vi "remote.Log In.vi"(0 "SLSC Remote in":refnum<class "SLSC Interface.lvclass">, 1 "username":string, 2 "password":string, 5 "chassis":refnum<k21>, 11 "error in (no error)":errorcluster, 12 "connect timeout (60 sec)":dbl=60.0, 13 "save credentials to disk? (F)":bool) -> (4 "SLSC Remote out":refnum<class "SLSC Interface.lvclass">, 15 "error out":errorcluster)   [LabVIEW 2016, in "SLSC Interfaces.lvlib" / "SLSC Interface.lvclass"]
uses:
  SLSC Interface Class/SLSC Interface.lvclass
  SLSC Interface Class/SLSC Interface.lvclass/SLSC Interface.ctl
  SLSC Interface Class/Read client handle.vi
  SLSC Interface Class/Read URL.vi
  <vilib>/NI/JSON Support for LabVIEW/JSON Data Classes/JSON Object/JSON Object.lvclass
  C:/Program Files (x86)/National Instruments/LabVIEW 2016/vi.lib/NI/JSON Support for LabVIEW/JSON Data Classes/JSON Datatype/JSON Null.lvclass
  SLSC Interface Class/Read session.vi
  <vilib>/NI/JSON Support for LabVIEW/JSON Data Classes/JSON Object/New JSON Object (Empty).vi
  <vilib>/NI/JSON Support for LabVIEW/JSON Data Classes/JSON Object/Insert Key Value Pair (Single String).vi
  <vilib>/NI/JSON Support for LabVIEW/JSON Data Classes/JSON Object/Insert Key Value Pair (Single Numeric).vi
  <vilib>/NI/JSON Support for LabVIEW/JSON Data Classes/JSON Object/Insert Key Value Pair (Single Boolean).vi
  <vilib>/NI/NI JSONRPC Server Framework/Classes/Server/Format Client Request (Auto-Increment).vi
  <vilib>/httpClient/POSTBuffer.vi
  <vilib>/NI/NI JSONRPC Server Framework/Classes/Server/Parse Response (Object).vi
  <vilib>/NI/NI JSONRPC Server Framework/Classes/Server/JSONRPC Server.lvclass
  <vilib>/httpClient/LabVIEWHTTPClient.lvlib
  <vilib>/NI/JSON Support for LabVIEW/JSON Data Classes/JSON Helper/JSON Helper.lvclass
  C:/Program Files (x86)/National Instruments/LabVIEW 2016/vi.lib/NI/JSON Support for LabVIEW/JSON Data Classes/JSON Structured Type/JSON Structure.lvclass
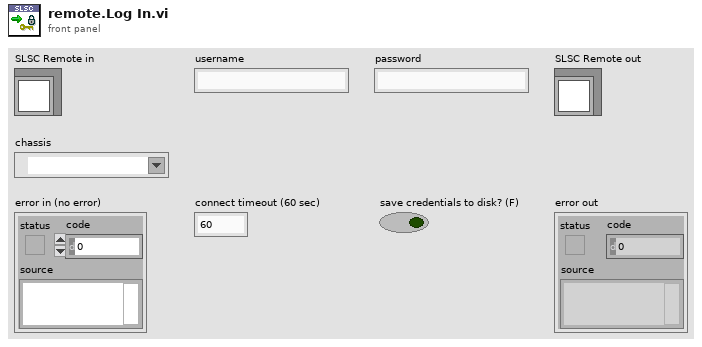
[diagram p1: front panel]
types:
  T1 = typedef "LabVIEWHTTPClient.lvlib/ClientHandle.ctl" = refnum<k1>
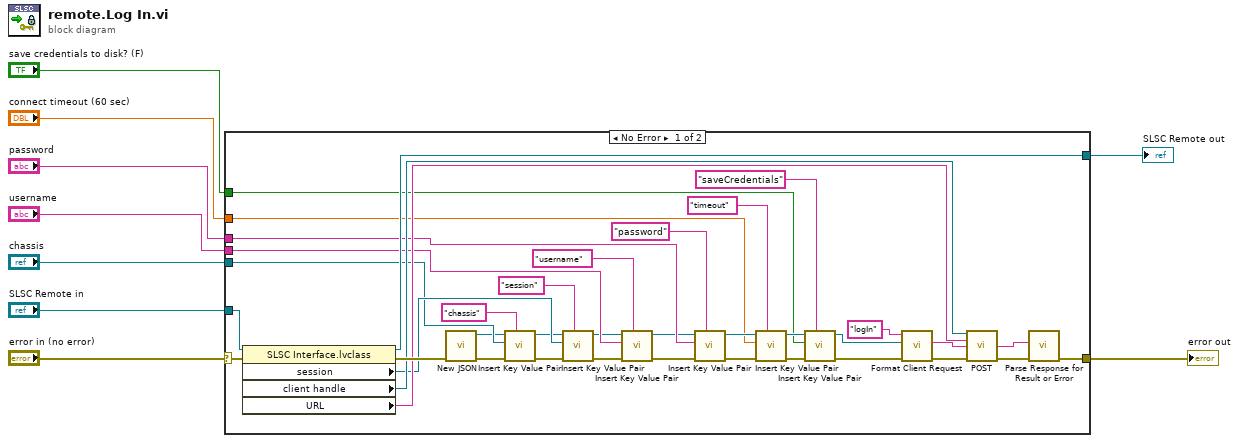
[diagram p0: block diagram]
diagram:
  n1 = case shown="No Error" "error in (no error)" {
    selector: "error in (no error)" -> [w45 w48]
    tunnel: "chassis" -> [w19 _]
    tunnel: "SLSC Remote in" -> [w47 w49]
    tunnel: [w46 w49] -> w5
    tunnel: [w34 w48] -> w6
    tunnel: "username" -> [w26 _]
    tunnel: "password" -> [w25 _]
    tunnel: "connect timeout (60 sec)" -> [w11 _]
    tunnel: "save credentials to disk? (F)" -> [w10 _]
    frame No Error {
      n2 = property class="SLSC Interface.lvclass"(reference=w47, error in=w45) -> (reference out=w46:refnum<class "SLSC Interface.lvclass">, error out=w44:errorcluster, "session"=w21:refnum<k21>, "client handle"=w39:T1, "URL"=w38:string)
      n3 = call-poly <vilib>:"New JSON.vi"("error in (no error)"=w44) -> ("error out"=w43:errorcluster, "JSON Object out"=w17:refnum<class "JSON Object.lvclass">)  [unwired: 9 in]
      n4 = call-poly <vilib>:"Insert Key Value Pair.vi"("key"="chassis" ("Name"), "error in (no error)"=w43, "value"=w19, "JSON Object in"=w17) -> ("error out"=w42:errorcluster, "JSON Object out"=w16:refnum<class "JSON Object.lvclass">)  [unwired: 5 in, 1 out]
      n5 = call-poly <vilib>:"Insert Key Value Pair.vi"("key"="session" ("Name"), "error in (no error)"=w42, "value"=w21, "JSON Object in"=w16) -> ("error out"=w33:errorcluster, "JSON Object out"=w15:refnum<class "JSON Object.lvclass">)  [unwired: 5 in, 1 out]
      n6 = call-poly <vilib>:"Insert Key Value Pair.vi"("key"="username" ("String"), "error in (no error)"=w33, "value"=w26, "JSON Object in"=w15) -> ("error out"=w32:errorcluster, "JSON Object out"=w14:refnum<class "JSON Object.lvclass">)  [unwired: 5 in, 1 out]
      n7 = call-poly <vilib>:"Insert Key Value Pair.vi"("key"="password" ("Name"), "error in (no error)"=w32, "value"=w25, "JSON Object in"=w14) -> ("error out"=w31:errorcluster, "JSON Object out"=w13:refnum<class "JSON Object.lvclass">)  [unwired: 5 in, 1 out]
      n8 = call-poly <vilib>:"Insert Key Value Pair.vi"("key"="timeout" ("Name"), "error in (no error)"=w31, "value"=w11, "JSON Object in"=w13) -> ("error out"=w30:errorcluster, "JSON Object out"=w12:refnum<class "JSON Object.lvclass">)  [unwired: 5 in, 1 out]
      n9 = call-poly <vilib>:"Insert Key Value Pair.vi"("key"="saveCredentials" ("Name"), "error in (no error)"=w30, "value"=w10, "JSON Object in"=w12) -> ("error out"=w27:errorcluster, "JSON Object out"=w28:refnum<class "JSON Object.lvclass">)  [unwired: 5 in, 1 out]
      n10 = call-poly <vilib>:"Format Client Request.vi"("error in (no error)"=w27, "JSON in"=w28, "method"="logIn") -> ("error out"=w37:errorcluster, "Request String"=w40:string)  [unwired: 7 in]
      n11 = call-poly <vilib>:"POST.vi"("client handle"=w39, "url"=w38, "buffer"=w40, "error in (no error)"=w37) -> ("body"=w36:string, "error out"=w35:errorcluster)  [unwired: 8 in, 2 out]
      n12 = call-poly <vilib>:"Parse Response for Result or Error.vi"("error in"=w35, "Response String In"=w36) -> ("error out"=w34:errorcluster)  [unwired: 7 in, 2 out]
    }
    frame Error {
    }
  }
  "error out" <- w6
  "SLSC Remote out" <- w5
